vi "To Variant.vi"(8 "Error In":errorcluster, 11 "TD Bool":refnum<class "Bool.lvclass">) -> (0 "Error Out":errorcluster, 2 "Variant":variant)   [LabVIEW 2017, in "Tree API.lvlib" / "Bool.lvclass"]
doc: "Dynamic dispatch interface for conversion of Tree Data classes to variant LV data."
uses:
  Bool.lvclass
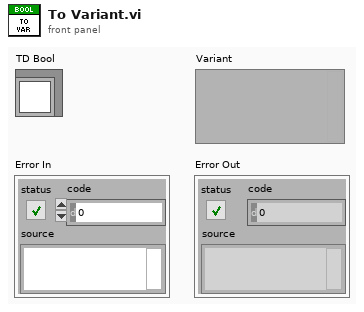
[diagram p1: front panel]
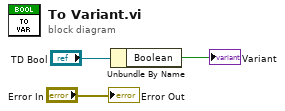
[diagram p0: block diagram]
diagram:
  n1 = Unbundle By Name("TD Bool") -> ("Boolean"=→"Variant":bool)
  "Error Out" <- "Error In"
